vi "Cryo-Con Get Configuration.vi"(8 "Error In":errorcluster, 10 "Config":T1={"Record Channels"=["A"], "Record raw signal"=FALSE, "Set point"=0.0, "Record heater"=FALSE, "Ramp rate"=0.0, "P"=0.0, "I"=0.0, "D"=0.0, "Control"=enum."Off", "P manual"=0.0, "Output #"=1}, 11 "VISA resource name":refnum<visa-resource-name>) -> (0 "Error Out":errorcluster, 2 "Config out":T1={"Record Channels"=["A"], "Record raw signal"=FALSE, "Set point"=0.0, "Record heater"=FALSE, "Ramp rate"=0.0, "P"=1.0, "I"=0.0, "D"=60.0, "Control"=enum."Off", "P manual"=0.0, "Output #"=0}, 3 "VISA resource name out":refnum<visa-resource-name>)   [LabVIEW 2021]
uses:
  Temperature Controller Driver/T controller configuration.ctl
  Temperature Controller/Controls/Control Mode.ctl
  GPIB/VISA  Send Receive.vi
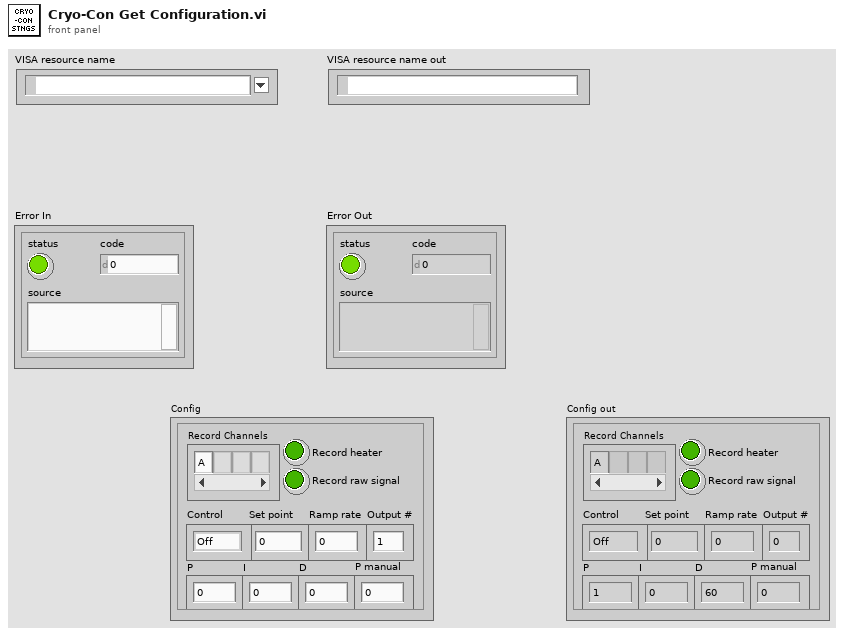
[diagram p1: front panel]
types:
  T1 = typedef "T controller configuration.ctl" = cluster{"Record Channels":string[], "Record raw signal":bool, "Set point":dbl, "Record heater":bool, "Ramp rate":dbl, "P":dbl, "I":dbl, "D":dbl, "Control":T2, "P manual":dbl, "Output #":i32}
  T2 = typedef "Control Mode.ctl" = enum16{"Off", "PID", "Ramp", "Manual", "Table"}
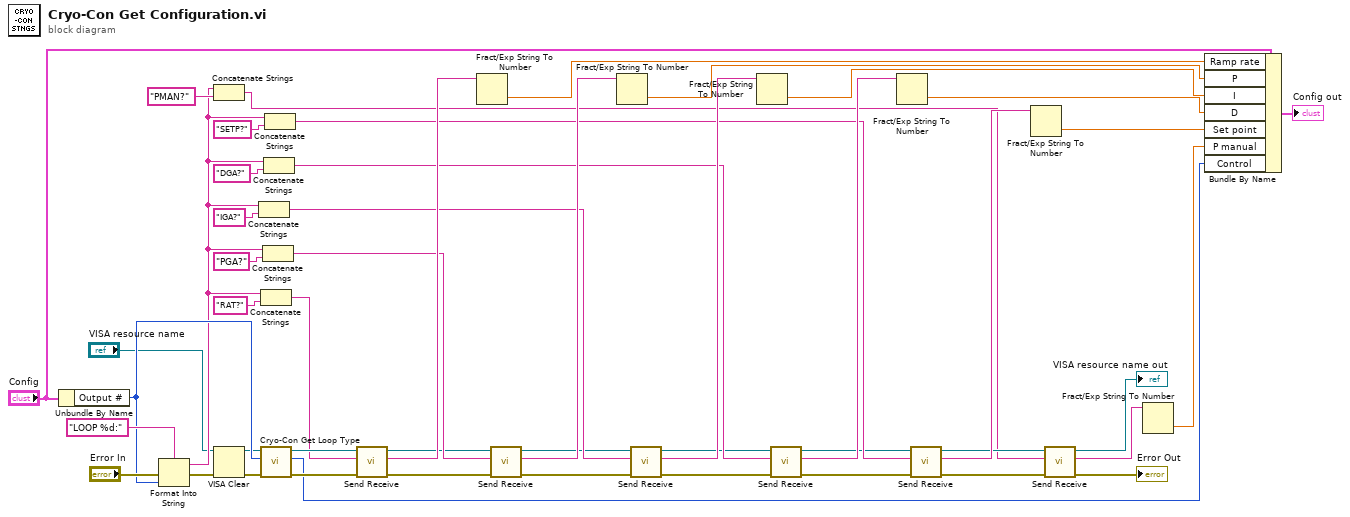
[diagram p0: block diagram]
diagram:
  n1 = Unbundle By Name("Config") -> ("Output #"=w22:i32)
  n2 = Format Into String(format string="LOOP %d:", error in="Error In", w22) -> (resulting string=w11:string, error out=w1:errorcluster)  [unwired: 1 in]
  n3 = Concatenate Strings(w11, "PMAN?" ("format string")) -> (w5:string)
  n4 = VISA Clear(VISA resource name="VISA resource name", error in (no error)=w1) -> (VISA resource name out=w3:refnum<visa-resource-name>, error out=w4:errorcluster)
  n5 = Concatenate Strings(w11, "IGA?" ("format string")) -> (w38:string)
  n6 = Concatenate Strings(w11, "RAT?" ("format string")) -> (w43:string)
  n7 = call "Cryo-Con Get Loop Type.vi"("error in (no error)"=w4, "Loop number"=w22, "VISA Resource Name"=w3) -> ("error out"=w48:errorcluster, "Set T"=w7:T2, "VISA Resource Name Out"=w49:refnum<visa-resource-name>)  [unwired: 6 in]
  n8 = Concatenate Strings(w11, "PGA?" ("format string")) -> (w39:string)
  n9 = Concatenate Strings(w11, "DGA?" ("format string")) -> (w33:string)
  n10 = Concatenate Strings(w11, "SETP?" ("format string")) -> (w26:string)
  n11 = call-poly "Send Receive.vi"("error in (no error)"=w48, "data string in"=w43, "VISA Resource Name"=w49) -> ("error out"=w41:errorcluster, "data string out"=w47:string, "VISA Resource Name Out"=w30:refnum<visa-resource-name>)  [unwired: 6 in]
  n12 = Fract/Exp String To Number(string=w47) -> (number=w20:dbl)  [unwired: 3 in, 1 out]
  n13 = call-poly "Send Receive.vi"("error in (no error)"=w41, "data string in"=w39, "VISA Resource Name"=w30) -> ("error out"=w32:errorcluster, "data string out"=w40:string, "VISA Resource Name Out"=w29:refnum<visa-resource-name>)  [unwired: 6 in]
  n14 = Fract/Exp String To Number(string=w40) -> (number=w19:dbl)  [unwired: 3 in, 1 out]
  n15 = call-poly "Send Receive.vi"("error in (no error)"=w32, "data string in"=w38, "VISA Resource Name"=w29) -> ("error out"=w31:errorcluster, "data string out"=w37:string, "VISA Resource Name Out"=w28:refnum<visa-resource-name>)  [unwired: 6 in]
  n16 = Fract/Exp String To Number(string=w37) -> (number=w18:dbl)  [unwired: 3 in, 1 out]
  n17 = call-poly "Send Receive.vi"("error in (no error)"=w31, "data string in"=w33, "VISA Resource Name"=w28) -> ("error out"=w23:errorcluster, "data string out"=w34:string, "VISA Resource Name Out"=w25:refnum<visa-resource-name>)  [unwired: 6 in]
  n18 = Fract/Exp String To Number(string=w34) -> (number=w17:dbl)  [unwired: 3 in, 1 out]
  n19 = call-poly "Send Receive.vi"("error in (no error)"=w23, "data string in"=w26, "VISA Resource Name"=w25) -> ("error out"=w13:errorcluster, "data string out"=w24:string, "VISA Resource Name Out"=w8:refnum<visa-resource-name>)  [unwired: 6 in]
  n20 = Fract/Exp String To Number(string=w24) -> (number=w15:dbl)  [unwired: 3 in, 1 out]
  n21 = call-poly "Send Receive.vi"("error in (no error)"=w13, "data string in"=w5, "VISA Resource Name"=w8) -> ("error out"=→"Error Out":errorcluster, "data string out"=w10:string, "VISA Resource Name Out"=→"VISA resource name out":refnum<visa-resource-name>)  [unwired: 6 in]
  n22 = Fract/Exp String To Number(string=w10) -> (number=w9:dbl)  [unwired: 3 in, 1 out]
  n23 = Bundle By Name(cluster="Config", "Ramp rate"=w20, "P"=w19, "I"=w18, "D"=w17, "Set point"=w15, "P manual"=w9, "Control"=w7) -> (→"Config out":T1)
